vi "Call Read Target ESI Files.vi"(8 "error in":errorcluster, 11 "IP address":string) -> (0 "error out":errorcluster, 3 "Existing Target Profiles":string[](array[string]))   [LabVIEW 2019, in "SEECD System Explorer.lvlib"]
uses:
  SEECD System Explorer.lvlib
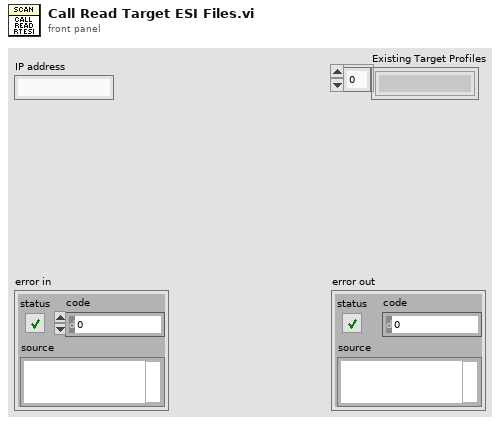
[diagram p1: front panel]
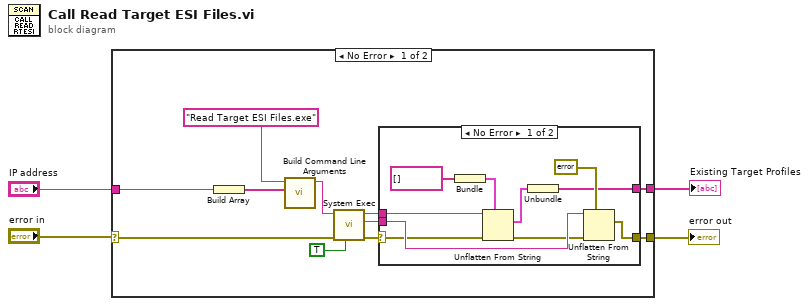
[diagram p0: block diagram]
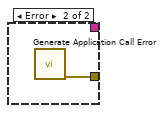
[diagram p2: hidden frame]
diagram:
  n1 = case shown="No Error" "error in" {
    selector: "error in" -> [w15 w27]
    tunnel: [w12 w27] -> w4
    tunnel: "IP address" -> [w7 _]
    tunnel: [w14 _] -> w1
    frame No Error {
      n2 = Build Array(w7) -> (w6:string[])
      n3 = call "Build Command Line Arguments.vi"("Arguments"=w6, "Executable File Name"="Read Target ESI Files.exe" ("name or relative path")) -> ("Command Line"=w5:string)  [unwired: 9 in]
      n4 = call <vilib>:"System Exec.vi"("run minimized? (F)"=TRUE, "error in (no error)"=w15, "command line"=w5) -> ("error out"=w13:errorcluster, "standard error"=w10:string, "standard output"=w11:string)  [unwired: 5 in, 1 out]
      n5 = case shown="No Error" w13 {
        selector: w13 -> [w22 _]
        tunnel: [w18 _] -> w14
        tunnel: [w24 w26] -> w12
        tunnel: w11 -> [w21 _]
        tunnel: w10 -> [w23 _]
        frame No Error {
          n6 = Bundle("Existing Target Profiles"=string[] []) -> (w20:cluster{"Existing Target Profiles":string[]})  [unwired: 1 in]
          n7 = Unflatten From String(type=w20, binary string=w21, error in (no error)=w22) -> (value=w19:cluster{"Existing Target Profiles":string[]}, error out=w17:errorcluster)  [unwired: 2 in, 1 out]
          n8 = Unbundle(w19) -> ("Existing Target Profiles"=w18:string[])
          n9 = Unflatten From String(type=errorcluster {"status"=FALSE, "code"=0, "source"=""} ("error in (no error)"), binary string=w23, error in (no error)=w17) -> (value=w24:errorcluster)  [unwired: 2 in, 2 out]
        }
        frame Error {
          n10 = call "Generate Application Call Error.vi"() -> ("error out"=w26:errorcluster)  [unwired: 11 in]
        }
      }
    }
    frame Error {
    }
  }
  "error out" <- w4
  "Existing Target Profiles" <- w1
